vi "Is VI in Memory.vi"(8 "error in (no error)":errorcluster, 9 "VI Path":path, 11 "All VIs in Memory":string[](array[string])) -> (0 "error out":errorcluster, 1 "VI ref out":refnum<vi>, 2 "Is VI in Memory":bool)   [LabVIEW 2020]
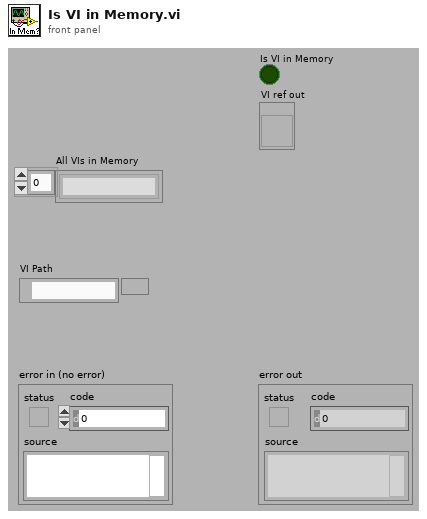
[diagram p1: front panel]
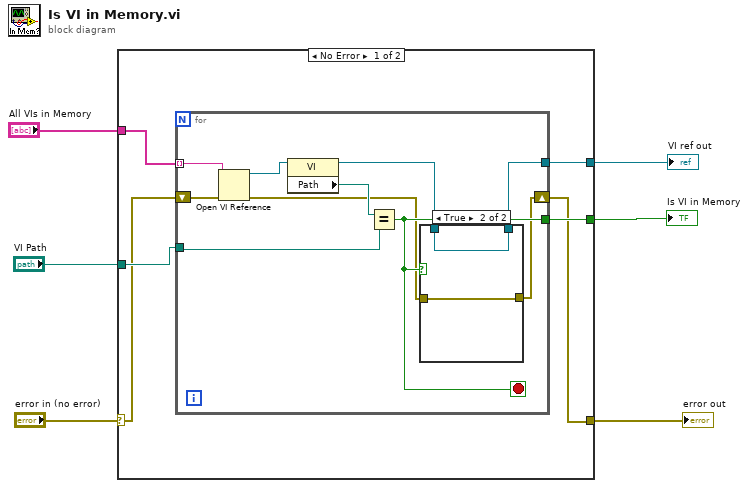
[diagram p0: block diagram]
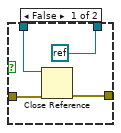
[diagram p2: hidden frame]
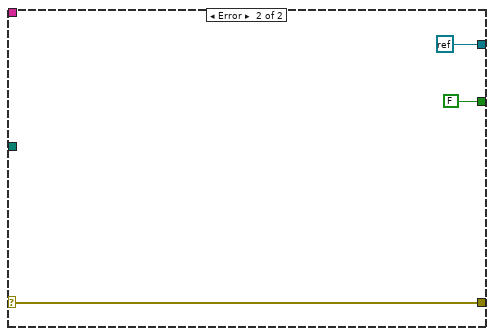
[diagram p3: hidden frame]
diagram:
  n1 = case shown="No Error" "error in (no error)" {
    selector: "error in (no error)" -> [w8 w31]
    tunnel: "All VIs in Memory" -> [w12 _]
    tunnel: [w7 w31] -> w4
    tunnel: "VI Path" -> [w11 _]
    tunnel: [w10 FALSE] -> w2
    tunnel: [w9 refnum<k0> refnum] -> w1
    frame No Error {
      n2 = for {
        tunnel: w12 -> [w22] mode=indexing
        shift-right: [w15] -> w7
        shift-left: w8 -> [w21]
        tunnel: w11 -> [w19]
        tunnel: [w17] -> w10
        tunnel: [w13] -> w9
        stop <- w17 stop-if-true
        n3 = Open VI Reference(vi path=w22, error in (no error)=w21) -> (vi reference=w20:refnum<vi>, error out=w16:errorcluster)  [unwired: 4 out]
        n4 = property class="VI"(reference=w20) -> (reference out=w14:refnum<vi>, "Path"=w18:path)  [unwired: 1 in, 1 out]
        n5 = Equal?(x=w18, y=w19) -> (x = y?=w17:bool)
        n6 = case shown="True" w17 {
          tunnel: w14 -> [w26 w28]
          tunnel: w16 -> [w25 w27]
          tunnel: [w24 w27] -> w15
          tunnel: [refnum<k0> refnum w28] -> w13
          frame False {
            n7 = Close Reference(reference=w26, error in (no error)=w25) -> (error out=w24:errorcluster)
          }
          frame True {
          }
        }
      }
    }
    frame Error {
    }
  }
  "error out" <- w4
  "Is VI in Memory" <- w2
  "VI ref out" <- w1
